vi "Write Remaining Data.vi"(8 "error in":errorcluster, 11 "cPAS Data in":refnum<class "cPAS Data.lvclass">) -> (0 "error out":errorcluster, 3 "cPAS Data out":refnum<class "cPAS Data.lvclass">)   [LabVIEW 2014, in "cPAS Data.lvclass"]
uses:
  cPAS Data.lvclass
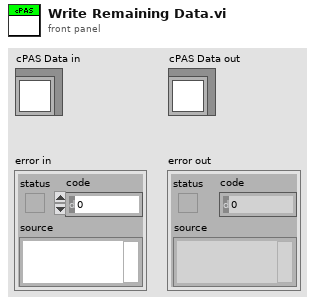
[diagram p1: front panel]
types:
  T1 = enum16{"big-endian, network order", "native, host order", "little-endian"}
  T2 = cluster{"24V":sgl, "+15V":sgl, "- 15V":sgl, "12V":sgl, "Aux Volt":sgl}
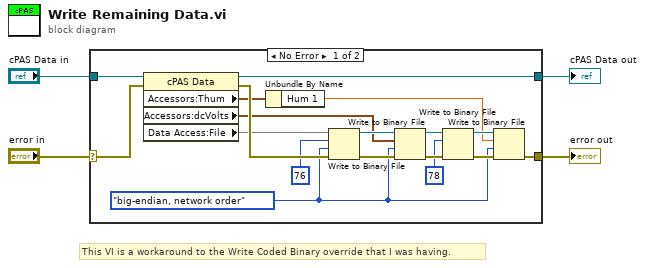
[diagram p0: block diagram]
diagram:
  # "This VI is a workaround to the Write Coded Binary override that I was having."
  n1 = case shown="No Error" "error in" {
    selector: "error in" -> [w8 w24]
    tunnel: [w7 w24] -> w3
    tunnel: [w9 w23] -> w1
    tunnel: "cPAS Data in" -> [w10 w23]
    frame No Error {
      w11 = T1."big-endian, network order" ("byte order (0:big-endian, network order)")
      n2 = property class="cPAS Data"(reference=w10, error in=w8) -> (reference out=w9:refnum<class "cPAS Data.lvclass">, error out=w22:errorcluster, "Accessors:Thum"=w6:cluster{"Hum 1":sgl, "Hum 2":sgl}, "Accessors:dcVolts"=w12:T2, "Data Access:File"=w13)
      n3 = Unbundle By Name(w6) -> ("Hum 1"=w5:sgl)
      n4 = Write to Binary File(file (use dialog)=w13, data=u8 76, error in=w22, 9:w11) -> (refnum out=w20:refnum<file>, error out=w19:errorcluster)  [unwired: 2 in, 1 out]
      n5 = Write to Binary File(file (use dialog)=w20, data=w12, error in=w19, 9:w11) -> (refnum out=w18:refnum<file>, error out=w17:errorcluster)  [unwired: 2 in, 1 out]
      n6 = Write to Binary File(file (use dialog)=w18, data=u8 78, error in=w17) -> (refnum out=w15:refnum<file>, error out=w14:errorcluster)  [unwired: 3 in, 1 out]
      n7 = Write to Binary File(file (use dialog)=w15, data=w5, error in=w14, 9:w11) -> (error out=w7:errorcluster)  [unwired: 2 in, 2 out]
    }
    frame Error {
    }
  }
  "error out" <- w3
  "cPAS Data out" <- w1
